vi "DLTS - setup pulse timing (SubVI).vi"(8 "error in (no error)":errorcluster, 9 "TUpulse off time":dbl=-1.0, 10 "TUpulse on time":dbl, 11 "Handle Out in":T1 {"Handle" format="0x%08x"; "Conn" format="0x%08x"}) -> (0 "error out":errorcluster, 3 "Handle Out out":T1 {"Handle" format="0x%08x"; "Conn" format="0x%08x"})   [LabVIEW 2019]
doc: "Configures DLTS biasing pulse timing"
uses:
  <instrlib>/Zurich Instruments LabOne/Public/ziTypeHandle.ctl
  <instrlib>/Zurich Instruments LabOne/Public/Configure/ziSetValueDoubleArray.vi
  <instrlib>/Zurich Instruments LabOne/Zurich Instruments LabOne.lvlib
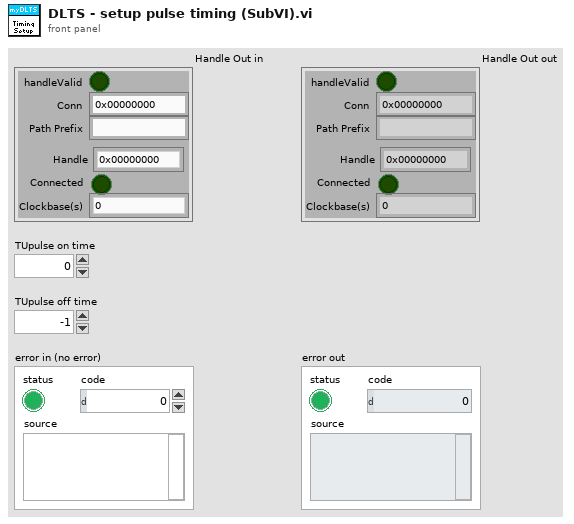
[diagram p1: front panel]
types:
  T1 = typedef "Zurich Instruments LabOne.lvlib/ziTypeHandle.ctl" = cluster{"handleValid":bool, "Conn":u64, "Path Prefix":string, "Handle":u64, "Connected":bool, "Clockbase(s)":dbl}
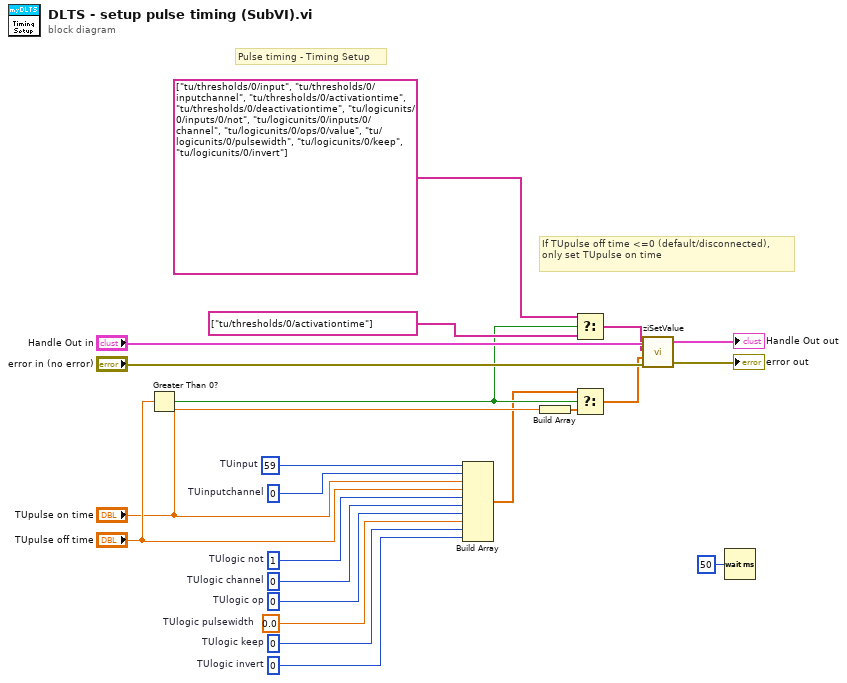
[diagram p0: block diagram]
diagram:
  w18 = 0  # TUlogic invert
  w17 = 0  # TUlogic keep
  w16 = 0.0  # TUlogic pulsewidth
  w15 = 0  # TUlogic op
  w14 = 0  # TUlogic channel
  w13 = 1  # TUlogic not
  w12 = 0  # TUinputchannel
  w11 = 59  # TUinput
  # "If TUpulse off time <=0 (default/disconnected), only set TUpulse on time"
  # "Pulse timing - Timing Setup"
  n1 = Greater Than 0?(x="TUpulse off time") -> (x > 0?=w6:bool)
  n2 = Build Array(w11, w12, "TUpulse on time", "TUpulse off time", w13, w14, w15, w16, w17, w18) -> (w3:dbl[])
  n3 = Build Array("TUpulse on time") -> (w5:dbl[])
  n4 = Select(t=string[] ["tu/thresholds/0/input", "tu/thresholds/0/inputchannel", "tu/thresholds/0/activationtime", "tu/thresholds/0/deactivationtime", "tu/logicunits/0/inputs/0/not", "tu/logicunits/0/inputs/0/channel", "tu/logicunits/0/ops/0/value", "tu/logicunits/0/pulsewidth", "tu/logicunits/0/keep", "tu/logicunits/0/invert"] ("Paths"), s=w6, f=string[] ["tu/thresholds/0/activationtime"]) -> (s? t:f=w7:string[])
  n5 = Select(t=w3, s=w6, f=w5) -> (s? t:f=w2:dbl[])
  n6 = call-poly <instrlib>:"ziSetValue.vi"("Error In"="error in (no error)", "Values"=w2, "Paths"=w7, "Handle In"="Handle Out in") -> ("Error Out"=→"error out":errorcluster, "Handle Out"=→"Handle Out out":T1)  [unwired: 1 in]
  n7 = Wait (ms)(milliseconds to wait=u32 50) -> ()  [unwired: 1 out]
